vi "TxP Measure.vi"(7 "Selector String":string, 8 "error in (no error)":errorcluster, 11 "Instrument Handle In":refnum<k21>) -> (0 "error out":errorcluster, 2 "TxP Results":T1 {"Minimum Power (dBm)" format="%.2f"; "Maximum Power (dBm)" format="%.2f"; "Peak to Average Ratio (dB)" format="%.2f"; "Average Mean Power (dBm)" format="%.2f"}, 3 "Instrument Handle Out":refnum<k21>)   [LabVIEW 2016, in "RFmxSpecAn.lvlib"]
uses:
  RFmxSpecAn.lvlib
  Typedefs/TxP Results.ctl
  <vilib>/RFmx/SpecAn/mx/RFmxSpecAn.llb/RFmxSpecAn Select Measurement (Single).vi
  <vilib>/RFmx/SpecAn/mx/RFmxSpecAn.llb/RFmxSpecAn TXP Fetch Power Trace.vi
  <vilib>/RFmx/SpecAn/mx/RFmxSpecAn.llb/RFmxSpecAn TXP Fetch Measurement.vi
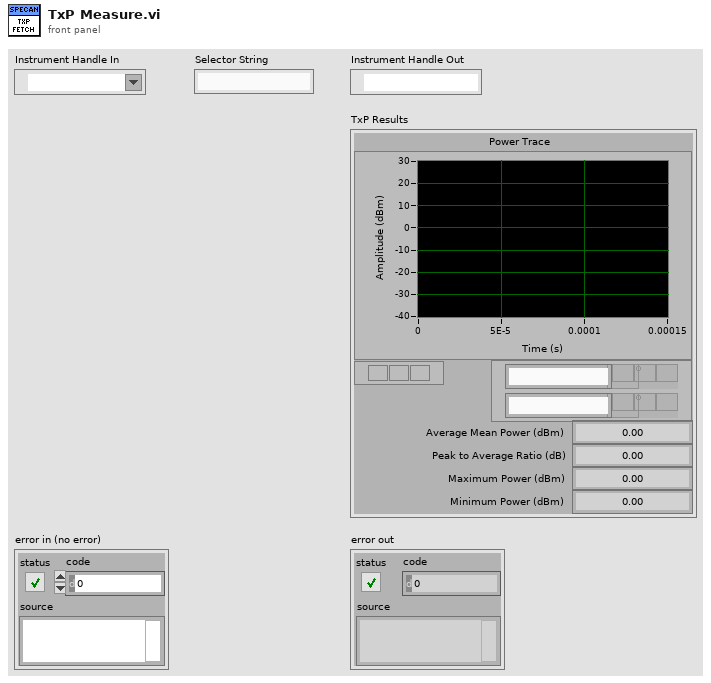
[diagram p1: front panel]
types:
  T1 = typedef "RFmxSpecAn.lvlib/TxP Results.ctl" = cluster{"Power Trace":cluster{"x0":dbl, "dx":dbl, "y":sgl[]}, "Average Mean Power (dBm)":dbl, "Peak to Average Ratio (dB)":dbl, "Maximum Power (dBm)":dbl, "Minimum Power (dBm)":dbl}
  T2 = enum16{"ACP", "CCDF", "CHP", "FCnt", "Harmonics", "OBW", "SEM", "Spectrum", "Spur", "TXP", "AMPM", "DPD", "IQ", "IM", "NF", "PhaseNoise"}
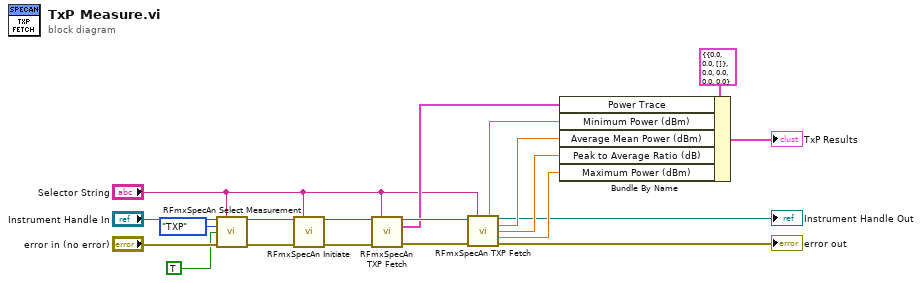
[diagram p0: block diagram]
diagram:
  n1 = call-poly <vilib>:"RFmxSpecAn Select Measurement.vi"("Instrument Handle In"="Instrument Handle In", "Selector String"="Selector String", "Measurement"=T2."TXP", "Enable All Traces"=TRUE, "error in (no error)"="error in (no error)") -> ("Instrument Handle Out"=w3:refnum<k21>, "error out"=w8:errorcluster)  [unwired: 9 in]
  n2 = call <vilib>:"RFmxSpecAn Initiate.vi"("Instrument Handle In"=w3, "Selector String"="Selector String", "error in (no error)"=w8) -> ("Instrument Handle Out"=w2:refnum<k21>, "error out"=w4:errorcluster)  [unwired: 10 in, 1 out]
  n3 = call-poly <vilib>:"RFmxSpecAn TXP Fetch.vi"("Instrument Handle In"=w2, "Selector String"="Selector String", "error in (no error)"=w4) -> ("Instrument Handle Out"=w20:refnum<k21>, "Power (dBm)"=w17:cluster{"x0":dbl, "dx":dbl, "y":sgl[]}, "error out"=w19:errorcluster)  [unwired: 10 in]
  n4 = call-poly <vilib>:"RFmxSpecAn TXP Fetch.vi"("Instrument Handle In"=w20, "Selector String"="Selector String", "error in (no error)"=w19) -> ("Minimum Power (dBm)"=w13:dbl, "Instrument Handle Out"=→"Instrument Handle Out":refnum<k21>, "Average Mean Power (dBm)"=w16:dbl, "Peak to Average Ratio (dB)"=w15:dbl, "Maximum Power (dBm)"=w14:dbl, "error out"=→"error out":errorcluster)  [unwired: 7 in]
  n5 = Bundle By Name(cluster=T1 {"Power Trace"={"x0"=0.0, "dx"=0.0, "y"=[]}, "Average Mean Power (dBm)"=0.0, "Peak to Average Ratio (dB)"=0.0, "Maximum Power (dBm)"=0.0, "Minimum Power (dBm)"=0.0} ("Cluster"), "Power Trace"=w17, "Minimum Power (dBm)"=w13, "Average Mean Power (dBm)"=w16, "Peak to Average Ratio (dB)"=w15, "Maximum Power (dBm)"=w14) -> (→"TxP Results":T1)
